vi "Read Registry.vi"(11 "ConfigurableActor in":refnum<class "ConfigurableActor.lvclass">) -> (2 "Registry":refnum<data-value>, 3 "ConfigurableActor out":refnum<class "ConfigurableActor.lvclass">)   [LabVIEW 2014, in "ConfigurableActor.lvclass"]
uses:
  ConfigurableActor.lvclass
  <vilib>/LabVIEW Open Source Project/Unicity/UniqueName/Registry/NameRegistry.lvclass
  ConfigurableActor.lvclass/ConfigurableActor.ctl
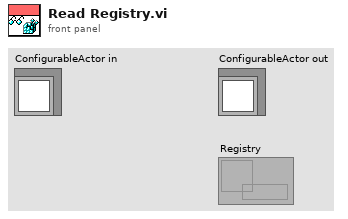
[diagram p1: front panel]
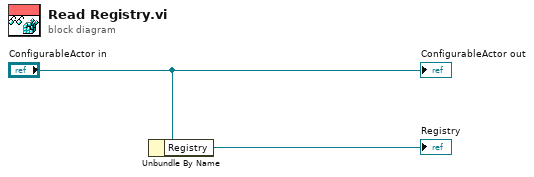
[diagram p0: block diagram]
diagram:
  n1 = Unbundle By Name("ConfigurableActor in") -> ("Registry"=→"Registry":refnum<data-value>)
  "ConfigurableActor out" <- "ConfigurableActor in"
